vi "DAQ.Create DAQmx Asynch Write.vi"(8 "error in (no error)":errorcluster, 11 "Array":refnum<k21>[](array[refnum])) -> (0 "error out":errorcluster, 3 "VI out":refnum<vi>)   [LabVIEW 2019, in "Instrument.Lockin.lvlib" / "Instrument.DAQ.lvclass"]
uses:
  Instrument.DAQ.lvclass
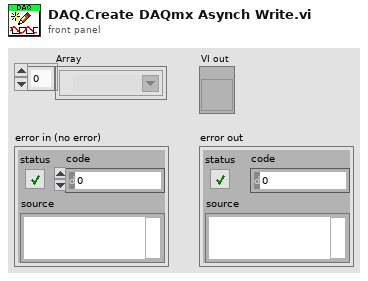
[diagram p1: front panel]
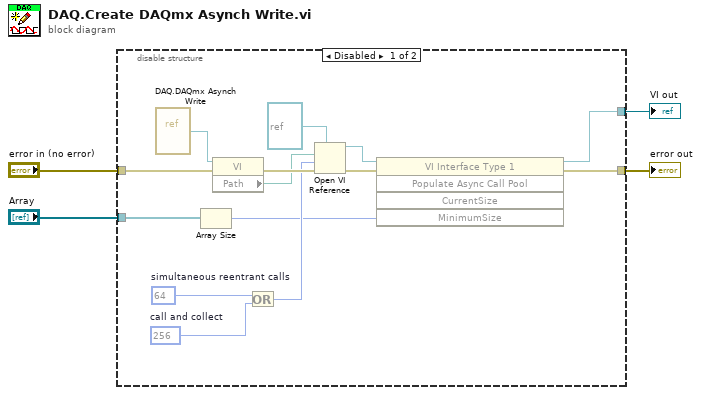
[diagram p0: block diagram]
diagram:
  n1 = disable-structure shown="Disabled" {
    disable-tunnel: [w13 _] -> w4
    disable-tunnel: "Array" -> [w9 _]
    disable-tunnel: [w8 w19] -> w2
    disable-tunnel: "error in (no error)" -> [w7 w19]
    frame Disabled {
      w11 = 64  # simultaneous reentrant calls
      w10 = 256  # call and collect
      n2 = vi-ref "DAQ.DAQmx Asynch Write.vi"() -> (w5:refnum<vi>)
      n3 = Array Size(array=w9) -> (size(s)=w6:i32)
      n4 = property class="VI"(reference=w5, error in=w7) -> (error out=w15:errorcluster, "Path"=w14:path)  [unwired: 1 out]
      n5 = Or(x=w11, y=w10) -> (x .or. y?=w12:i32)
      n6 = Open VI Reference(type specifier VI Refnum (for type only)=refnum<vi> refnum, vi path=w14, options=w12, error in (no error)=w15) -> (vi reference=w17:refnum<vi>, error out=w18:errorcluster)  [unwired: 2 in]
      n7 = invoke class="VI Interface Type 1" method="Populate Async Call Pool"(reference=w17, error in=w18, "MinimumSize"=w6) -> (reference out=w13:refnum<vi>, error out=w8:errorcluster)  [unwired: 2 in, 3 out]
    }
    frame Enabled {
    }
  }
  "VI out" <- w4
  "error out" <- w2
